vi "SimpleVoltageCurrentCapture.vi"() -> ()   [LabVIEW 2014]
uses:
  <vilib>/Utility/error.llb/DialogType.ctl
  <vilib>/DAQmx/write.llb/DAQmx Write (Analog Wfm 1Chan NSamp).vi
  <vilib>/DAQmx/read.llb/DAQmx Read (Analog 1D Wfm NChan NSamp).vi
  <vilib>/DAQmx/create/channels.llb/DAQmx Create Channel (AI-Voltage-Basic).vi
  <vilib>/DAQmx/configure/timing.llb/DAQmx Timing (Sample Clock).vi
  <vilib>/DAQmx/create/channels.llb/DAQmx Create Channel (AO-Voltage-Basic).vi
  <vilib>/DAQmx/miscellaneous.llb/DAQmx Fill In Error Info.vi
  <vilib>/measure/matone.llb/Extract Single Tone Information 1 Chan.vi
  <vilib>/measure/madcrms.llb/Basic Averaged DC-RMS for 1 Chan.vi
  <vilib>/addons/Electrical Power/Basic/Measurement/Power (1 Channel).vi
  <vilib>/imath/engines/lvmath2/RunTimeEngine/Managers/WorkSpace/UID Generator.vi
  <vilib>/imath/engines/lvmath2/RunTimeEngine/BuiltInFunctions/abs/NIMS_abs(signed).vi
  <instcachedir>/0/NIMS_abs(signed)_C4FCB8E6058B49B797C7C8D53CA5F6EC.lvgen/NIMS_abs(signed)_C4FCB8E6058B49B797C7C8D53CA5F6EC_000.vi
  <vilib>/imath/engines/lvmath2/RunTimeEngine/RunTimeType/NIMS_RunTimeType_From StrictType (excl LVString).vi
  <instcachedir>/0/NIMS_RunTimeType_From StrictType (excl LVString)_15A5391EEA9C4AACB9955AC755B83D29.lvgen/NIMS_RunTimeType_From StrictType (excl LVString)_15A5391EEA9C4AACB9955AC755B83D29_000.vi
  <vilib>/imath/engines/lvmath2/RunTimeEngine/LocalVariableDefStatement/MC_LocalVariableDefStatement_Display.vi
  <vilib>/imath/engines/lvmath2/RunTimeEngine/Managers/SymbolTable/Clear UID.vi
  <vilib>/imath/engines/lvmath2/RunTimeEngine/NodeEndStatement/NIMS_NodeEndStatement_Output.vi
  <instcachedir>/0/NIMS_NodeEndStatement_Output_53EC0D466D134D7ABD903AC30B43404B.lvgen/NIMS_NodeEndStatement_Output_53EC0D466D134D7ABD903AC30B43404B_001.vi
  <vilib>/imath/engines/lvmath2/RunTimeEngine/ErrorHandling/NIMS_Finalize Error.vi
  <vilib>/measure/NI_MAPro.lvlib
  <resource>/objmgr/daqmx.rc
  <vilib>/imath/engines/lvmath2/RunTimeEngine/Managers/SymbolTable/NIMS_WorkSpace.lvlib
  <vilib>/Analysis/NI_AALPro.lvlib
  <vilib>/addons/Electrical Power/Basic/NI_EP_Basic.lvlib
panel:
  out "Numeric":i32
  out "output":waveform(dbl)(graph)={"t0"=timestamp(329.7 s since 1904-01-01), "dt"=0.0001, "Y"=array[998 elements]}
  in  "Triger Pulse":bool
  out "real pulse duration":dbl=0.0005
  in  "Pulse Amplitude":dbl=5.0
  in  "Pulse Duration (s)":dbl=0.0005
  out "Pulse":bool
  out "External Command":string="{ \"command\" : \"ac_v\", \"value\" : 0.0 }\n"
  out "TCP Control":bool
  in  "TCP command in port":u16=37086
  out "IV read duration actual (ms)":dbl=96.66666666666667
  out "IV read duration (ms)":dbl=100.0
  in  "Electrode mode":bool
  out "TCP ADC":bool
  out "Last Transmited Loop Id":i32=-1
  out "Read Loop Id":i32=3296
  out "AC Voltage":dbl=0.015165725599678053 format="%0.2p"
  out "AC Current":dbl=0.0011066504587498834 format="%0.2p"
  in  "TCP data out port":u16=37085
  out "AC I_in amplitude chart":dbl(graph)=0.0011066504587498834
  out "I_in RMS":dbl(graph)=19.597394261114836
  out "Power plot":dbl(graph)=-1.7020442408267042
  out "Phase difference plot":dbl(graph)=291.4389580733613
  out "I _in Power Spectrum":T1(graph)={0.0, "df"=10.000000000000007, "Power Spectrum (V^2 rms)"=[384.05781864212213, 1.2812941664551393e-08, 1.2802014188361118e-07, 4.812511296015439e-09, 3.4604865493181385e-09, 8.59844797514965e-08, 1.540100486406839e-08, 2.7635332673585536e-08, 2.0089632622951103e-07, 2.5397753546698656e-08, 3.0209073625980115e-08, 5.243292855206259e-08, 2.7564168394443787e-08, 1.3099304476836114e-08, 1.0159404130224844e-07, 8.76543417641275e-09, 2.276381425075035e-08, 4.6904899271181916e-09, 9.941137463137335e-09, 1.2446977421983896e-08, 8.579209932008616e-08, 2.0104817814097586e-10, 1.8991275344229937e-08, 9.837888338792514e-08, 6.481034062706947e-08, 7.925498497472071e-08, 7.731911747461447e-08, 1.5782095489234225e-09, 3.279570790933137e-08, 1.349939768318964e-07, 9.63615092297605e-09, 2.9275372363938947e-08, 1.3176389712752455e-07, 4.018791844757954e-08, 3.8489049210479654e-08, 3.209664549280304e-08, 6.31520653319137e-08, 1.062910830558792e-07, 9.767664666009403e-08, 3.7143944529906357e-09, 8.1056328458131e-09, 5.178062053483344e-08, 5.679670399970084e-08, 1.907727598794696e-08, 9.69946931205068e-09, 3.5621842812701156e-08, 3.555275859885974e-08, 1.99230098156712e-07, 5.369362919485012e-08, 4.1863615058039905e-08, 1.2338652677581583e-08, 4.697281997314641e-08, 3.993580605238427e-08, 1.70035079391051e-08, 1.6594795089805326e-08, 1.516958186684704e-07, 7.575946548396981e-08, 2.5612321514999438e-08, 5.2738297712080446e-08, 1.1590760683173937e-07, 2.0944189064547272e-08, 1.0264229746821111e-07, 6.978167227192961e-08, 1.1508175740867062e-07, 8.093287052603338e-08, 3.1301731540051725e-08, 1.454693917268169e-08, 2.9108329285014653e-08, 2.409433105650876e-07, 3.459793455758188e-08, 7.532687221251975e-09, 1.2005768049469254e-08, 4.634528439936204e-08, 1.6745745681336807e-08, 6.172958760008946e-08, 9.655445431991258e-08, 2.4918781782308413e-08, 1.3380696016198607e-08, 9.273295644922437e-09, 9.384676050914868e-09, 5.045622969104436e-08, 1.328983752516565e-07, 1.1221780541437274e-07, 4.141449358779783e-08, 2.903977936074104e-08, 3.8537967200709724e-09, 4.708037887736474e-08, 8.291494602872388e-08, 7.70570911232849e-08, 1.966098960787566e-07, 4.534805900984656e-09, 1.726199435323091e-08, 3.3680113687564556e-08, 1.3805146619739584e-08, 3.472836601578071e-08, 2.630915209312157e-08, 8.168496626292698e-08, 5.0623868146713205e-09, 1.115875074934071e-07, 1.7741127446006096e-07, 4.368995406929392e-08, 3.2021447596937008e-09, 3.48779398152876e-08, 3.081985764940028e-08, 1.1096457286070956e-07, 4.60849417995993e-08, 3.779434226378727e-08, 4.347888166225807e-08, 1.6373452915251257e-09, 1.8808612179755276e-08, 7.988124958811374e-08, 4.376230558771452e-09, 3.339685828609752e-08, 1.0891895570542552e-07, 4.1536321590750644e-08, 4.8098653195030446e-08, 4.6601247081840685e-08, 8.391058107643042e-08, 1.0431839897374635e-08, 1.5214232021995607e-08, 1.8688923087010836e-07, 8.659765798597669e-08, 1.4491551422316902e-07, 2.141816801173361e-08, 1.2072901470805195e-09, 6.3913451504969056e-09, 2.2794143843174313e-08, 8.064368559082834e-08, 1.915399388627138e-07, 1.206705846213626e-08, 4.033054884196688e-09, 2.1342371658332653e-09, 6.075018915623819e-08, 1.4852245888680382e-07, 4.88419660733143e-09, 4.088409395652448e-08, 1.4026863668695995e-07, 2.2252630941062042e-07, 3.5832058304485996e-08, 2.3936499810289502e-08, 2.9039314574844087e-09, 2.3973293286931087e-08, 1.5836479233915926e-07, 2.23325561613219e-08, 1.696949460470778e-08, 8.26262872042607e-09, 6.50783217445291e-08, 1.0775111733297002e-08, 1.0390218139538638e-08, 1.3560599946394992e-08, 5.206753303012184e-08, 4.773172547667066e-09, 1.4873562740571618e-08, 1.9868712281171172e-08, 2.0981036336581242e-09, 8.945525119636087e-09, 4.0189259502991666e-08, 3.952424418931359e-08, 2.894034445292779e-08, 4.6490878327638985e-08, 4.524556389012339e-08, 1.2629162546160513e-09, 2.708985273619554e-08, 1.0223761490440988e-07, 3.594586961713648e-08, 3.5426269882768174e-08, 4.137147998757457e-08, 2.9552957073705045e-08, 2.3365565701057763e-08, 9.26388932893052e-08, 1.1109103449455194e-07, 3.409307933526586e-09, 1.2146773701920775e-07, 4.584882861390524e-08, 9.354375969972158e-08, 1.4321296597243922e-08, 5.977699519636451e-08, 5.9461219291895514e-08, 4.215040396774052e-08, 1.728463184328385e-08, 3.136769765310978e-08, 3.4377428728288975e-08, 4.8818253276382846e-08, 1.7013235743670174e-09, 9.447022422313127e-08, 5.75966470002399e-08, 1.127651177182249e-08, 7.27729417865729e-08, 1.856704451103715e-08, 4.948908503771827e-08, 1.983889196727655e-08, 5.10381999791832e-09, 1.5679008689252454e-08, 2.1741073758842818e-08, 3.7297112056119515e-08, 7.661161766255485e-08, 6.433430558102816e-08, 1.2813926302545611e-08, 3.600763990317574e-07, 1.4561070888716884e-08, 4.949647036914003e-08, 8.129625906523154e-08, 2.9420403092238935e-09, 5.554047301193506e-09, 1.7827901643730115e-08, 1.504997723559743e-08, 1.5023578029496108e-07, 1.4670282386484361e-08, 2.28388341349861e-07, 2.5117787388135496e-08, 2.740953183198227e-08, 5.497198046704744e-08, 4.362641518031774e-08, 4.237109609144519e-08, 3.2688284362417267e-08, 2.5498427822612962e-08, 1.2520509050448536e-07, 2.233767041481571e-08, 3.2941470086808166e-08, 7.455358270842485e-09, 6.632980299635733e-08, 5.90896912581073e-08, 1.5304394394886514e-08, 5.3934963622971515e-08, 3.2767245686984146e-08, 9.612385712461888e-08, 4.8826354287495546e-08, 1.240211384939601e-07, 1.1460957546451582e-07, 2.4898905168286042e-09, 1.772980921047333e-08, 1.2385457753213336e-08, 4.9078691491580206e-08, 3.278255307059739e-08, 3.750081644919358e-09, 1.3931200494654658e-08, 5.444352857635511e-08, 6.546747175751133e-08, 1.711208662881434e-08, 1.929493601896497e-08, 3.6398341900996806e-08, 4.2966173465561364e-08, 3.6755869616760876e-08, 3.0176788219327757e-09, 3.011950207355472e-08, 3.512689585829536e-08, 2.8423326392118875e-08, 1.0022518357393645e-07, 1.4680561564719452e-08, 3.649625294637584e-08, 4.031497162692909e-08, 3.212272725614469e-08, 1.2139641391960006e-09, 7.021303894753625e-08, 3.3063149986789023e-09, 1.2393920457988236e-08, 1.0791191385073534e-08, 9.053090999153262e-08, 1.319342590437711e-07, 1.4614565189317268e-07, 1.5278657963461335e-10, 4.5527749043547795e-08, 1.452004595136674e-07, 1.664928120564626e-08, 5.140611957930399e-09, 7.727909612291312e-09, 1.6165225384853362e-08, 6.759152536161556e-08, 1.6398993135795582e-07, 5.630261658395028e-09, 2.5996461043004046e-08, 7.226217514336062e-09, 2.9198395761224226e-08, 4.306174983650763e-08, 7.004299924871136e-08, 3.519309319534001e-09, 2.91242462930489e-08, 7.060805187155125e-08, 8.056344362369779e-08, 6.180589372203309e-08, 6.940038681131413e-08, 1.1166596987411668e-08, 6.924308293151698e-08, 7.001606609260729e-08, 8.224478674786695e-08, 1.3951863080363851e-08, 2.1019018313440102e-08, 6.907251718509267e-08, 5.681299872508286e-09, 1.7677978248220832e-08, 2.6384605682949153e-08, 6.974791105187748e-09, 8.744045551935272e-08, 6.245895633033074e-08, 2.3706613961085087e-08, 5.624962818699386e-08, 2.8832627632170862e-08, 1.042337329119717e-09, 2.5334040670312715e-08, 2.434183685492577e-08, 7.86786715205878e-09, 1.6131885884860795e-08, 9.67930212416229e-08, 8.995733591895769e-08, 3.593948638488143e-08, 1.2541696411160845e-08, 9.554155040825989e-08, 1.7212725928829574e-08, 4.339613421388269e-08, 1.4565190207604182e-08, 7.578403908246223e-08, 3.723807576887632e-08, 2.2365903775075548e-08, 9.856433197334754e-09, 1.2901973481063502e-09, 3.237236539707619e-08, 1.3401762776921863e-08, 4.28802900320129e-08, 1.009290130906903e-07, 1.1396783394352265e-08, 2.531839857522575e-09, 4.3163400538895804e-08, 8.202540043777047e-08, 8.05816149377029e-09, 1.993864670886027e-08, 1.3644193500555042e-08, 1.3710128091232536e-07, 1.2638350417317973e-07, 5.7553454709946467e-08, 2.5779488948016492e-08, 3.547853169452205e-08, 1.927531482405474e-08, 2.1686066535790113e-08, 5.705752181882103e-08, 3.872519367448343e-08, 2.5710443279786668e-08, 2.745824248594476e-08, 1.0053202733111108e-08, 1.420870517456479e-07, 1.3291045114345208e-07, 1.5089874386483102e-08, 1.3383166408501238e-08, 4.7639242285258216e-08, 4.2779638261412625e-08, 3.5198664594141145e-08, 4.70674751344519e-08, 1.5640362866699093e-08, 2.777259741109804e-08, 1.8464546583383468e-07, 3.5526622377151104e-08, 6.992173052859764e-08, 7.04500361147302e-08, 2.317990914179313e-07, 8.160084189023287e-08, 3.800938308072212e-08, 9.045009934960116e-08, 1.2123057541864966e-07, 9.378510145173343e-09, 9.410955336235093e-08, 3.263838524099404e-08, 3.5637629667962905e-09, 4.77995455931702e-08, 5.368568140428507e-08, 1.322668580298105e-07, 1.0525664473288381e-08, 4.2409000894338724e-08, 1.1913821826190874e-07, 3.6223643278452168e-09, 2.9364053248634797e-08, 6.802727007201526e-08, 2.4686475295655384e-08, 1.3865394342703764e-07, 7.448398837323908e-08, 3.088265147226928e-08, 8.276128342601035e-08, 2.8119971146810945e-09, 6.5311068330998e-08, 8.246058705122179e-08, 1.9612968776879275e-07, 8.688316194537927e-08, 1.0572137449711188e-07, 1.4978541326265806e-08, 7.220451672668149e-09, 3.539964837407443e-08, 4.508792174056677e-08, 1.667337014738283e-08, 7.250899914777877e-08, 6.79692735908802e-08, 2.640801847008435e-08, 8.403841705833863e-09, 3.368100306159142e-08, 4.9455949186695094e-09, 9.330160576087414e-08, 9.1280438659868e-09, 6.971658854059668e-08, 1.9278804379235124e-08, 8.85741070762139e-09, 6.550471987073927e-08, 3.820630276229358e-08, 2.687291584215985e-08, 2.3908490507636175e-08, 2.321404069218755e-08, 3.2214778162993593e-08, 4.388028386243561e-08, 1.2882393967833918e-08, 6.7536187752439464e-09, 1.1744915357741611e-07, 7.18914884229133e-08, 1.9895175149726103e-07, 3.2400929572333717e-09, 9.297016272154701e-08, 9.934642824917249e-08, 8.321767937785236e-08, 5.670142195274526e-08, 4.951672860997498e-08, 1.8452713170003762e-08, 5.4116149816271593e-08, 2.0809817958948804e-08, 2.6881821288426383e-08, 2.1190492285073913e-08, 5.47989710922767e-08, 4.578562112689227e-08, 5.334322628142155e-08, 2.48547407773874e-08, 6.866572229520074e-09, 7.3369066098468025e-09, 1.1056786439640651e-08, 3.2700412463793237e-09, 2.0075139460641065e-08, 2.3881469546759143e-08, 8.966300203801532e-09, 1.2809432909660115e-07, 3.331679010715642e-08, 4.306759826704191e-08, 1.2583136041369329e-08, 7.012631803409424e-09, 4.3090819051484345e-09, 4.1692195154994595e-08, 2.6816404245670878e-08, 2.055791968326877e-09, 1.3672465345410637e-08, 2.1322010842748506e-08, 1.7596748428903714e-07, 4.4949830972338244e-08, 1.0341561615247105e-09, 2.9084161413310027e-08, 5.374387988786714e-08, 5.3349698825652904e-08, 1.4128611673613282e-09, 3.8801402600612375e-08, 3.109126241976239e-08, 3.1098370373565677e-10, 2.926361272648796e-08, 1.0898175300612959e-07, 4.075335025512814e-08, 1.335596727884363e-08, 1.062338525009548e-07, 3.232462556489928e-08, 8.387463408086883e-08, 1.2095210893322399e-08, 5.45334503104955e-08, 6.993509675464793e-08, 1.5871236299946294e-08, 2.706339141278551e-08, 3.0075189364169905e-09, 1.0028254063447421e-07, 3.277337661996945e-08, 5.1868628358504955e-08, 9.293476084725768e-08, 9.769168343283154e-09, 2.706819927179853e-08, 2.4966227555830077e-08, 8.834113407472588e-08, 6.397827295092539e-08, 8.372402954614174e-08, 8.712366376138589e-08, 7.078032696757265e-08, 2.7721920832500157e-08, 2.0649870212633134e-08, 2.5616407575308477e-08, 3.630868795735885e-08, 5.3707571062058424e-08, 8.275253292117417e-08, 1.2025549414428655e-08, 2.816125366723839e-08, 1.9186971038008822e-08, 3.6065289353871736e-11, 3.077636615403747e-09, 1.2370255816695734e-08, 1.0754168043709105e-07, 1.2675781071772376e-08, 2.898987401047185e-08, 4.473663379246382e-09, 3.3432293379785746e-08, 4.291579540032761e-08, 2.4535696702101412e-08, 1.7904473506491875e-08, 1.2969337345251354e-08, 3.579713233883194e-08, 8.306977329479662e-09, 1.1878600002587436e-08, 4.559792218223604e-11, 8.669398160192331e-08, 1.5443681894492246e-08, 5.7040102798961895e-08, 1.5455294911454466e-07, 2.2609903226912203e-08, 3.433387559706304e-08, 3.5888217413332686e-08, 1.941087982577279e-09, 2.7888395771837493e-08, 1.3803208628908935e-08, 4.9739989771947375e-08, 6.56012888081166e-09, 2.6591919552228713e-09, 6.630477591387785e-08, 1.3514257595649928e-07, 8.873512189501864e-09, 5.383031118323386e-09, 4.5274595599770835e-08, 1.2447679041540927e-07, 4.0434634444370015e-08, 6.3588242155244805e-09, 4.11760048095076e-09, 4.268369816964896e-09, 3.3258099950921486e-08, 2.6777423955798133e-08, 1.4054579830603142e-08, 1.156496532066109e-07, 3.395223102219717e-08, 6.230963112132895e-09, 1.3417625574245126e-08, 2.393050690932955e-07, 9.312228370000481e-09, 1.522541587312519e-08, 1.699491322214352e-08, 1.458984318693044e-07, 1.4460492208640573e-08, 1.835723265304928e-08, 2.3116603349858304e-08, 2.289455799857778e-08, 5.494128163325584e-09, 1.2559273977983916e-09, 8.723516991111303e-09, 9.56016883450206e-10, 1.5131137297979946e-08, 3.522116163379456e-08, 1.2780902906619467e-08, 2.0521225464484514e-08, 4.9710476866549016e-08, 2.6723133698770964e-09, 6.611761157113771e-08, 2.17822791711475e-07, 3.529362622749032e-08, 3.559740380027698e-08, 3.0236899652022443e-08, 9.880896042276115e-09, 1.653928219393416e-08, 2.2042260585923302e-08, 1.2119349725733237e-09, 4.263896438113567e-08, 5.9149398327904576e-08, 1.8856320402723333e-09, 2.281966109681429e-08, 5.754600253341904e-08, 5.0430552608468136e-08, 7.281465448753168e-09, 1.0395847299244066e-07, 1.924722587487483e-09, 1.695799004691539e-08, 2.6679578279876708e-08, 8.867086963010186e-09, 3.9524439443566215e-08, 1.1091448657235346e-07, 4.190708095098228e-09, 9.657150920733476e-08, 5.668301325774216e-09, 6.786300981728324e-08, 1.3223520082514987e-08, 3.404814354670106e-08, 4.223834658514782e-08, 3.8092545585383834e-08, 2.9289426487155407e-08, 1.0530287208659933e-09, 1.131762267293828e-09, 4.114102244117353e-08, 7.427298812970256e-09, 7.994081603306406e-08, 2.307637249031202e-07, 8.47724353652218e-09, 6.847887534885516e-08, 3.770997494988641e-08, 6.376403576558253e-08, 7.673744978583936e-09, 3.0838536546473044e-09, 4.700581307275506e-08, 1.3697280597830137e-07, 1.1261535051452766e-08, 5.3237899849287214e-08, 1.3605562050271097e-08, 2.2632883810616355e-08, 3.467444062765444e-08, 9.684926131445288e-08, 1.0635383763208542e-08, 4.356006403351025e-08, 2.2292295215612967e-07, 2.9470228128304294e-08, 2.875211386257933e-08, 2.041494292362725e-07, 6.39615845040027e-08, 5.977660555367681e-09, 6.26720749668346e-09, 5.984571161881243e-08, 1.2241633622245034e-07, 4.039287306691826e-08, 5.467584915815582e-09, 4.927474715376204e-08, 9.735781985113371e-08, 1.3217509024118545e-08, 3.3687734175546405e-08, 1.0542365775903405e-07, 4.517158944115068e-09, 9.726950682807576e-08, 2.387697232191287e-08, 2.7575186808995993e-08, 4.6071486658325546e-08, 8.41553900421575e-09, 1.6977322771610884e-08, 1.097823680664256e-07, 6.098758529615711e-09, 6.257708163733645e-08, 3.3555986343451286e-09, 8.692060193608496e-08, 4.468331572970971e-08, 6.390357629481517e-09, 2.6259264712257616e-08, 6.6745767634947644e-09, 3.587115148670567e-08, 3.523706140447217e-08, 4.126006093083413e-08, 2.4398341308567406e-08, 2.840067155681719e-09, 6.614688931874879e-09, 6.978648377097303e-08, 1.1478053355986801e-07, 4.073691886026624e-08, 6.4493241299896534e-09, 3.7683440704147226e-08, 3.0846089194508202e-09, 1.8048287772729807e-08, 3.337806676761065e-08, 2.977472660181094e-09, 1.0719164896676073e-07, 3.2536992415786914e-08, 2.2247660177635246e-08, 1.1476736545919476e-07, 2.8933953016947526e-08, 2.064106548584373e-08, 3.7223643656169426e-09, 1.843286134032916e-08, 1.892681922314445e-08, 3.712199947459135e-09, 1.6695753023392334e-08, 3.3218032569735317e-09, 1.6706432251667378e-08, 2.7067232095953743e-08, 3.837805045664525e-08, 1.1619197367608606e-07, 4.9924179949261114e-08, 8.464384625585008e-08, 9.690586418497523e-09, 7.179583796338114e-09, 6.217634841721696e-08, 3.2937274120486434e-08, 6.387779642630158e-08, 1.8470753266750935e-08, 3.5434607470527096e-08, 8.154309779516997e-08, 3.8727475603592855e-08, 1.0199854591655693e-08, 4.2154686318987e-08, 2.3675515842321936e-08, 6.333797743041275e-08, 8.985223681037249e-08, 6.497841644804245e-08, 2.914188943128051e-08, 4.560784310819312e-08, 1.3420003396361156e-08, 2.900222042456837e-08, 5.1518128797144566e-08, 3.0436935461941626e-08, 4.934019455520264e-09, 5.471322364342871e-08, 1.8294146250360306e-08, 1.0414336013540128e-07, 6.09864340420173e-09, 2.92160425235546e-08, 6.33802995592567e-08, 2.3095568168877672e-08, 2.428623669085022e-08, 2.5474306923772344e-08, 1.4080727261370552e-08, 4.5730253266045205e-08, 1.482467936763585e-08, 9.136500270332283e-08, 3.830435326792223e-08, 9.189028310552746e-08, 1.6171056084457597e-08, 2.6566605210262435e-08, 3.561591387341651e-10, 1.1896556157900548e-08, 1.3103660240603911e-08, 9.215464274720214e-08, 5.860820049635159e-09, 1.6596173016718347e-08, 7.999763077500574e-09, 2.754185521944779e-09, 4.64402722896503e-08, 4.2607496442374204e-10, 5.7640684496696686e-09, 2.4692578535470032e-08, 1.0675485918539571e-07, 5.075488929402043e-08, 4.316460162997264e-08, 5.0328599887739335e-09, 1.5668634672419503e-08, 1.0516052118361708e-07, 2.32509591277423e-09, 2.4635165122359574e-09, 1.583375293010504e-08, 6.084983597675616e-08, 2.453644347913616e-08, 4.3701545919628674e-08, 1.9314605782062944e-08, 2.649684168940553e-09, 4.777686684066642e-08, 2.65642672299213e-08, 8.31033371125199e-09, 4.481639519392982e-09, 3.0178667227519526e-08, 2.2981288156274775e-08, 7.140154264778307e-08, 3.4722699769530815e-08, 5.704763715175978e-09, 1.751524211308479e-08, 2.1017087512336967e-08, 1.988870949402694e-09, 4.735352048969542e-08, 1.0184723992817028e-08, 1.0817985812319281e-07, 7.937617084550854e-09, 4.390171603002758e-08, 2.4249724354616005e-08, 6.71845512229682e-09, 2.380422799459253e-08, 3.501038985542707e-09, 8.899732893447905e-09, 7.61403441167404e-09, 1.1723064942209228e-08, 2.2535947445598375e-08, 5.3283341740886406e-08, 9.105882842766771e-08, 3.3729411059946585e-08, 4.3940267301023304e-08, 2.1774650147897275e-08, 1.7759675438106559e-09, 2.3164876314791638e-08, 8.82667737460953e-08, 7.920169590988872e-08, 1.457761286773177e-09, 1.498315248699009e-08, 7.069854837264057e-08, 8.418069222277153e-08, 3.3678870417317805e-08, 3.1637243848242373e-08, 6.397428397409701e-09, 3.460972408839841e-08, 9.55072908342938e-09, 3.855474842185562e-08, 4.822523574453309e-09, 8.576037029797383e-08, 2.216732732464861e-08, 1.0731731417077834e-08, 3.361911636226198e-08, 4.434785797278945e-08, 1.3149154938533514e-07, 7.085277617290867e-08, 1.3224332278328078e-08, 1.9284574364398894e-09, 2.4047033269657476e-08, 1.0768520697283966e-07, 1.7553608393402726e-08, 1.3109152689706874e-07, 2.807246107263378e-08, 1.096355836380659e-07, 3.955468560380751e-09, 3.006742765984348e-08, 4.060701567467407e-08, 2.426992353465244e-08, 4.749588183834099e-08, 3.054592303261189e-08, 5.270269009564928e-08, 1.9402090796816506e-07, 2.5981880696136016e-09, 5.5230500003331466e-08, 4.64428118203972e-08, 2.1409958294161802e-10, 2.288066203188495e-08, 4.9980825755820055e-08, 1.674232052066761e-08, 5.6795402906730866e-08, 4.4322727225029266e-08, 2.0615649731299158e-08, 7.224529568663976e-08, 2.8688147683281023e-08, 3.402929380102517e-08, 3.141634728403987e-08, 1.7358690033472963e-08, 3.133749417697372e-08, 1.0551277143603665e-08, 9.12262312148022e-09, 1.2263549613662365e-07, 7.851780105651865e-09, 3.882878845776116e-08, 1.6315378053715675e-08, 4.51897149442903e-08, 4.781910596707131e-08, 8.756918742205452e-09, 1.1619690170861289e-07, 1.3626447576593534e-08, 1.0466638043043739e-08, 4.481027922250179e-08, 6.619337613530257e-08, 4.891485332269246e-10, 5.021283819602683e-10, 2.8838057047061665e-08, 8.830466536655001e-08, 1.1384736417596889e-08, 7.6499005222322e-08, 2.9832437883927726e-08, 2.417383384128457e-08, 1.0785370136026602e-07, 7.010394634407974e-08, 2.2124162123321894e-09, 5.1773802221779206e-08, 1.3397532270908865e-08, 2.9126431058974736e-08, 4.758678297839971e-09, 1.4859726717958443e-08, 9.579290796896566e-10, 8.382410500470574e-08, 7.080310312553315e-09, 2.7269490700317792e-09, 3.78099506757096e-08, 2.2906553673914697e-08, 4.958157328070189e-08, 1.277758260512456e-07, 1.5496214788254566e-08, 8.399442991850865e-09, 2.0974383688651131e-10, 7.653814131921521e-08, 1.0629574548079339e-07, 2.766875061154353e-07, 4.7209301917957004e-08, 1.1853201114255108e-07, 6.937763799420605e-08, 1.943847211188159e-08, 1.2681629635338865e-08, 7.171993830343981e-08, 7.3958949077661664e-09, 1.580972972534488e-08, 4.987889256805363e-09, 1.5029071415743658e-07, 1.1168613268630692e-07, 4.842068320148151e-08, 2.8670743014069843e-08, 7.552634389872825e-09, 3.55254938629143e-09, 4.690651654555333e-08, 9.617146907054903e-08, 3.94990254100245e-08, 2.7489632549819656e-08, 2.023782404563175e-08, 1.582435662631923e-09, 3.1974873935959875e-08, 7.579308377126686e-08, 2.7394549112873103e-08, 6.670929337086143e-08, 2.2152275059967488e-08, 1.3600706174955887e-08, 8.642822088262854e-09, 1.6107839488244233e-08, 8.781916880881347e-09, 3.097308817856408e-09, 2.4331582751704115e-08, 6.087922156947291e-09, 5.591098530859275e-08, 1.5982979887672207e-08, 9.264901077036059e-09, 2.0318992127978495e-09, 4.7404658141317465e-09, 9.173930614178918e-08, 7.152799793383632e-09, 4.131337501520023e-08, 1.2321417755982251e-08, 7.903663090317008e-09, 7.611818940957837e-09, 7.990165836186578e-09, 8.012796359838227e-08, 2.5157892757339584e-08, 6.415511471668318e-08, 1.243422988770215e-08, 3.49275645642184e-08, 3.863971064859102e-08, 3.1525505084313803e-08, 5.879145668430913e-08, 3.061627893242176e-10, 2.0131851195834646e-08, 1.7290712355540862e-08, 6.655802688588835e-08, 6.867426372189385e-09, 2.175498026467824e-08, 3.005946190978901e-08, 1.0725539817075016e-07, 9.906682015982944e-09, 1.9790589684394564e-08, 8.327225304946475e-10, 4.82468904336366e-08, 7.692639511651834e-09, 3.170008967763013e-08, 3.066931712221607e-08, 3.4791852466532265e-08, 3.10052077096927e-08, 4.901097856833149e-08, 8.408839697239916e-08, 1.418586799530674e-08, 4.7117279291701356e-08, 2.310797157029537e-09, 1.4445746485114266e-08, 6.164582516458707e-08, 2.5586830180460847e-08, 8.43785099374807e-08, 7.356410892271902e-08, 2.1885505924809696e-09, 4.7113911161041374e-08, 4.529500492545696e-08, 7.411155338885586e-08, 1.8176061752414404e-08, 5.47078902877339e-09, 3.892521506606838e-10, 2.374747848250165e-08, 3.062240367602707e-08, 6.296928503327405e-08, 4.056519728153538e-08, 5.6650512775013824e-08, 2.7827017241309587e-09, 4.078240649430459e-08, 3.2910104358428584e-10, 1.0526504712502214e-07, 9.78174397904926e-10, 1.8058767377346493e-08, 1.997747703478305e-09, 4.490674360637365e-08, 1.378005989277269e-08, 1.624907623861366e-07, 3.4692154033791618e-09, 5.161169405968163e-08, 2.285652862117089e-08, 8.639929263472041e-08, 7.931550118063889e-09, 1.4958674207442694e-08, 1.7480323340141855e-08, 7.60715363663814e-09, 2.6841314471108995e-08, 6.105837010272096e-08, 8.853220821608051e-09, 6.405650907048701e-11, 5.1875936854683124e-08, 5.3487242573330204e-08, 3.0559786850250324e-08, 3.981132646282874e-08, 1.8316925521886576e-08, 9.894007164716781e-09, 5.745944411915238e-09, 1.1143621083510306e-07, 6.238823250824436e-08, 5.541522312654942e-08, 4.3326359896416684e-09, 5.566996620276415e-08, 7.342344959134149e-09, 4.6455232860503546e-08, 4.237100632416493e-08, 1.1083885687882875e-08, 3.466333511838009e-08, 1.2120668315412319e-08, 4.6398686364235566e-08, 1.0906465242535382e-07, 1.1452052680285153e-09, 2.2273214276086914e-08, 1.753520472587311e-08]}
  out "phase difference":dbl=291.4389580733613
  out "detected frequency U":dbl=3135.969897018442 format="%.2p"
  out "detected frequency I":dbl=3776.0681138056098 format="%.2p"
  out "Cuurent and Voltage":waveform(dbl)[](graph)=[{"t0"=timestamp(3525370740.881266 s since 1904-01-01), "dt"=4.999999999999997e-05, "Y"=array[2000 elements], "attributes"=variant("NI_ChannelName"=variant(string "DAC/ai0"), "NI_UnitDescription"=variant(string "Volts"))}, {"t0"=timestamp(3525370740.881277 s since 1904-01-01), "dt"=4.999999999999997e-05, "Y"=array[2000 elements], "attributes"=variant("NI_ChannelName"=variant(string "DAC/ai1"), "NI_UnitDescription"=variant(string "Volts"))}]
  in  "Wave On/Off":bool
  in  "V_out":dbl
  out "Pulse generator":waveform(dbl)(graph)={"t0"=timestamp(329.7 s since 1904-01-01), "dt"=0.0001, "Y"=array[998 elements]}
  in  "V_out Units":dbl=0.01
  out "Mode Changed":bool
  out "V_out sampling rate":dbl=10000.0
  in  "Number of Samples":i32=1000
  out "Wave generator":waveform(dbl)(graph)={"t0"=timestamp(329.7 s since 1904-01-01), "dt"=0.0001, "Y"=array[1000 elements]}
  in  "Oscilator\nSettings":T2={"Waveform Type"=0, "Amplitude"=0.0, "Frequency"=50.0} {"Frequency" format="%0.2p"; "Amplitude" format="%0.2p"; "Waveform Type" items=["Sine Wave", "Triangle Wave", "Square Wave", "Sawtooth Wave"]}
  in  "V_out offset auto-calibrate":bool
  in  "V_out scaling auto-calibrate":bool
  in  "V_in scaling":dbl=1.0
  in  "I_in scaling":dbl=1.0
  in  "V_out offset":dbl
  in  "V_out scaling":dbl=1.0
  out "DC I_in Chart":dbl(graph)=19.59739315934959
  out "Closing Program":bool=TRUE
  in  "IV min V":dbl=-50.0
  in  "IV max V":dbl=50.0
  out "IV progress":dbl(slide)=1.0 scale=0.0..1.0
  in  "IV Relaxation Time (ms)":i32=1000 min=2 step=1
  in  "IV Number of Steps":i32=11 min=2 step=1
  in  "Take IV":bool
  out "Gain (alpha*beta)":dbl=0.1
  out "DC Voltage":dbl=-0.08685133420839247 format="%0.2p"
  out "DC Current":dbl=19.59739315934959 format="%0.2p"
  in  "Samples to read":i32=2000
  in  "I_in Units":dbl=1.0 caption="I Measured Scaling"
  in  "V_in Units":dbl=100.0
  in  "STOP":bool
  in  "Sampling frequency":dbl=20000.0 format="%#_6p"
  # "Units: \nVoltage [mV]\nCurrent [nA]"
  # "Configuration"
  # "Unit Config (don't change)"
  # "Calibration"
  # "Hz"
  # "delete?"
  # "TCP connection"
  # "Electrode Mode"
  # "Imaging"
  # "Deposition"
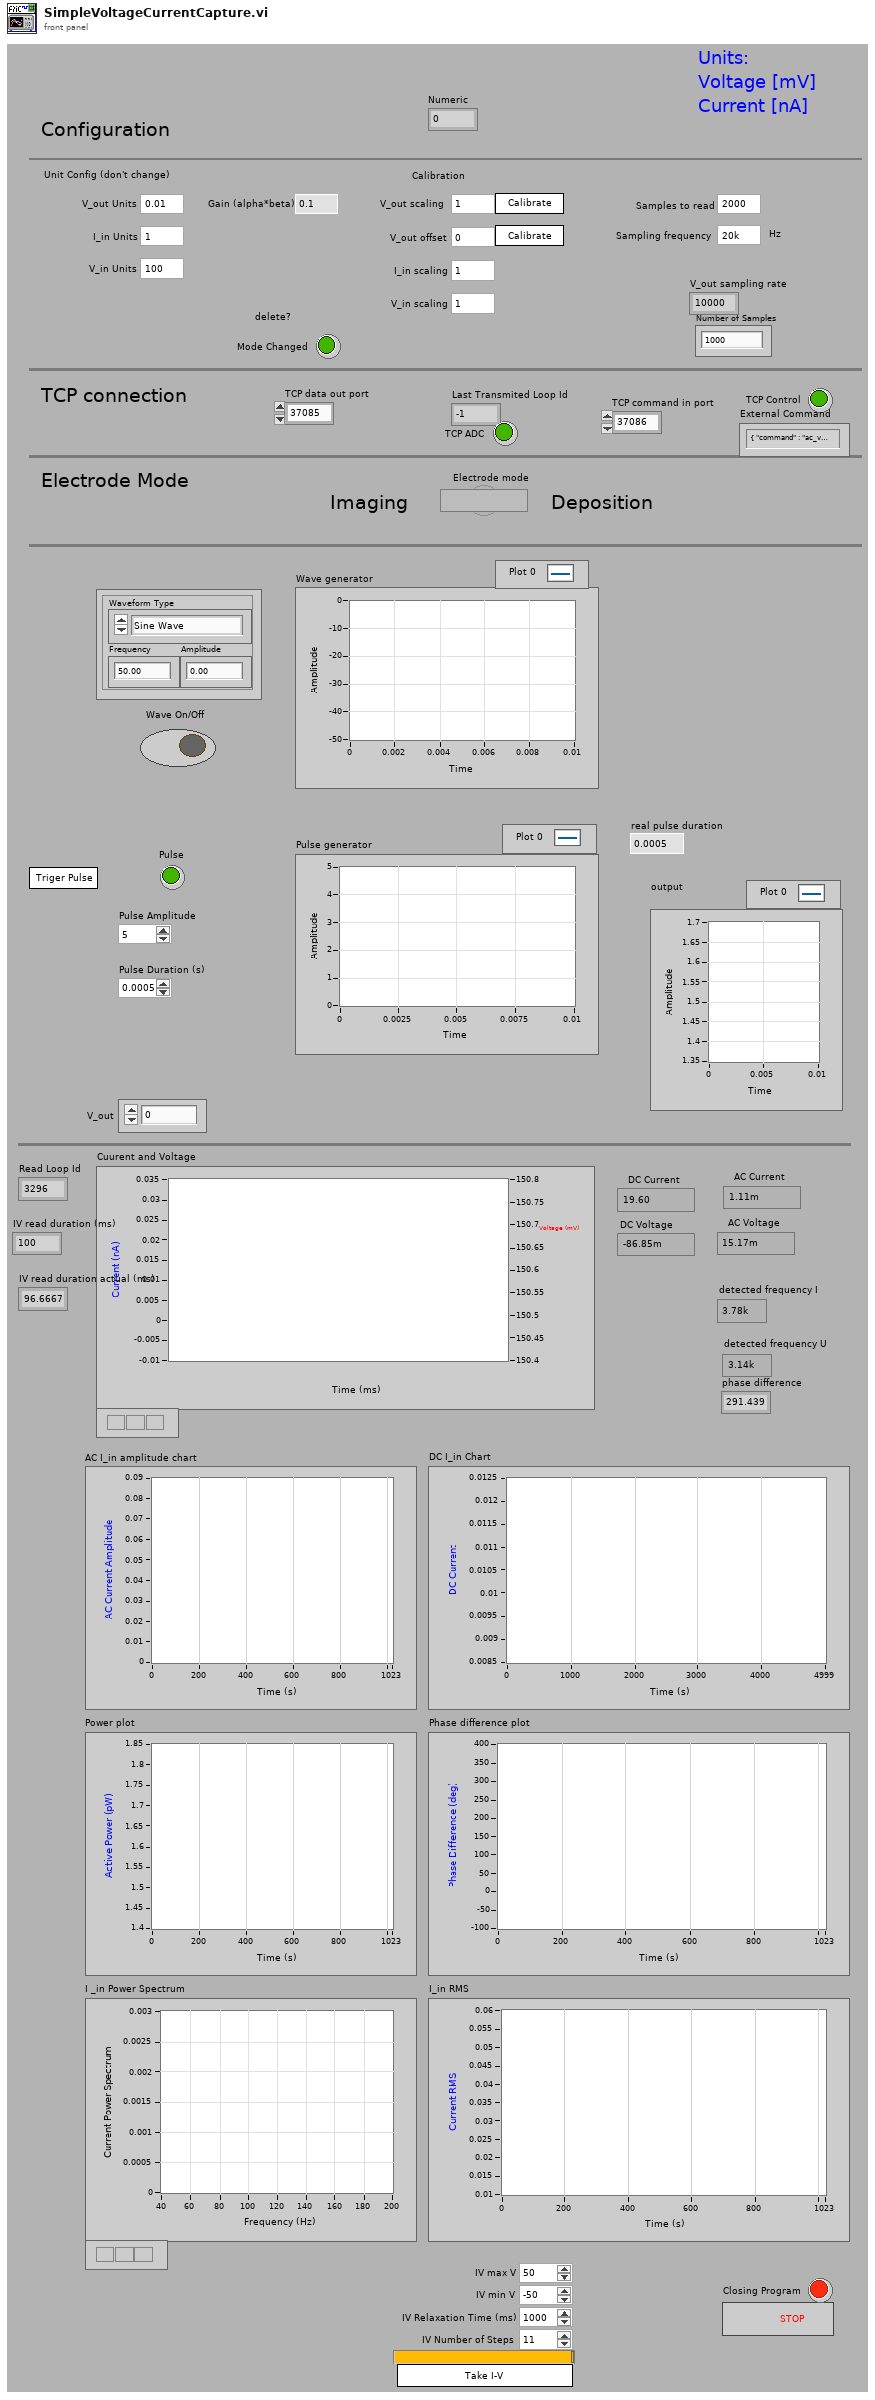
[diagram p1: front panel]
types:
  T1 = cluster{dbl, "df":dbl, "Power Spectrum (V^2 rms)":dbl[]}
  T2 = cluster{"Waveform Type":u16, "Amplitude":dbl, "Frequency":dbl}
  T3 = typedef "DialogType.ctl" = u16
  T4 = typedef "NI_EP_Basic.lvlib/basic_Power Value.ctl" = cluster{"active power [W]":dbl, "apparent power [VA]":dbl, "reactive power [VAR]":dbl, "power factor":dbl}
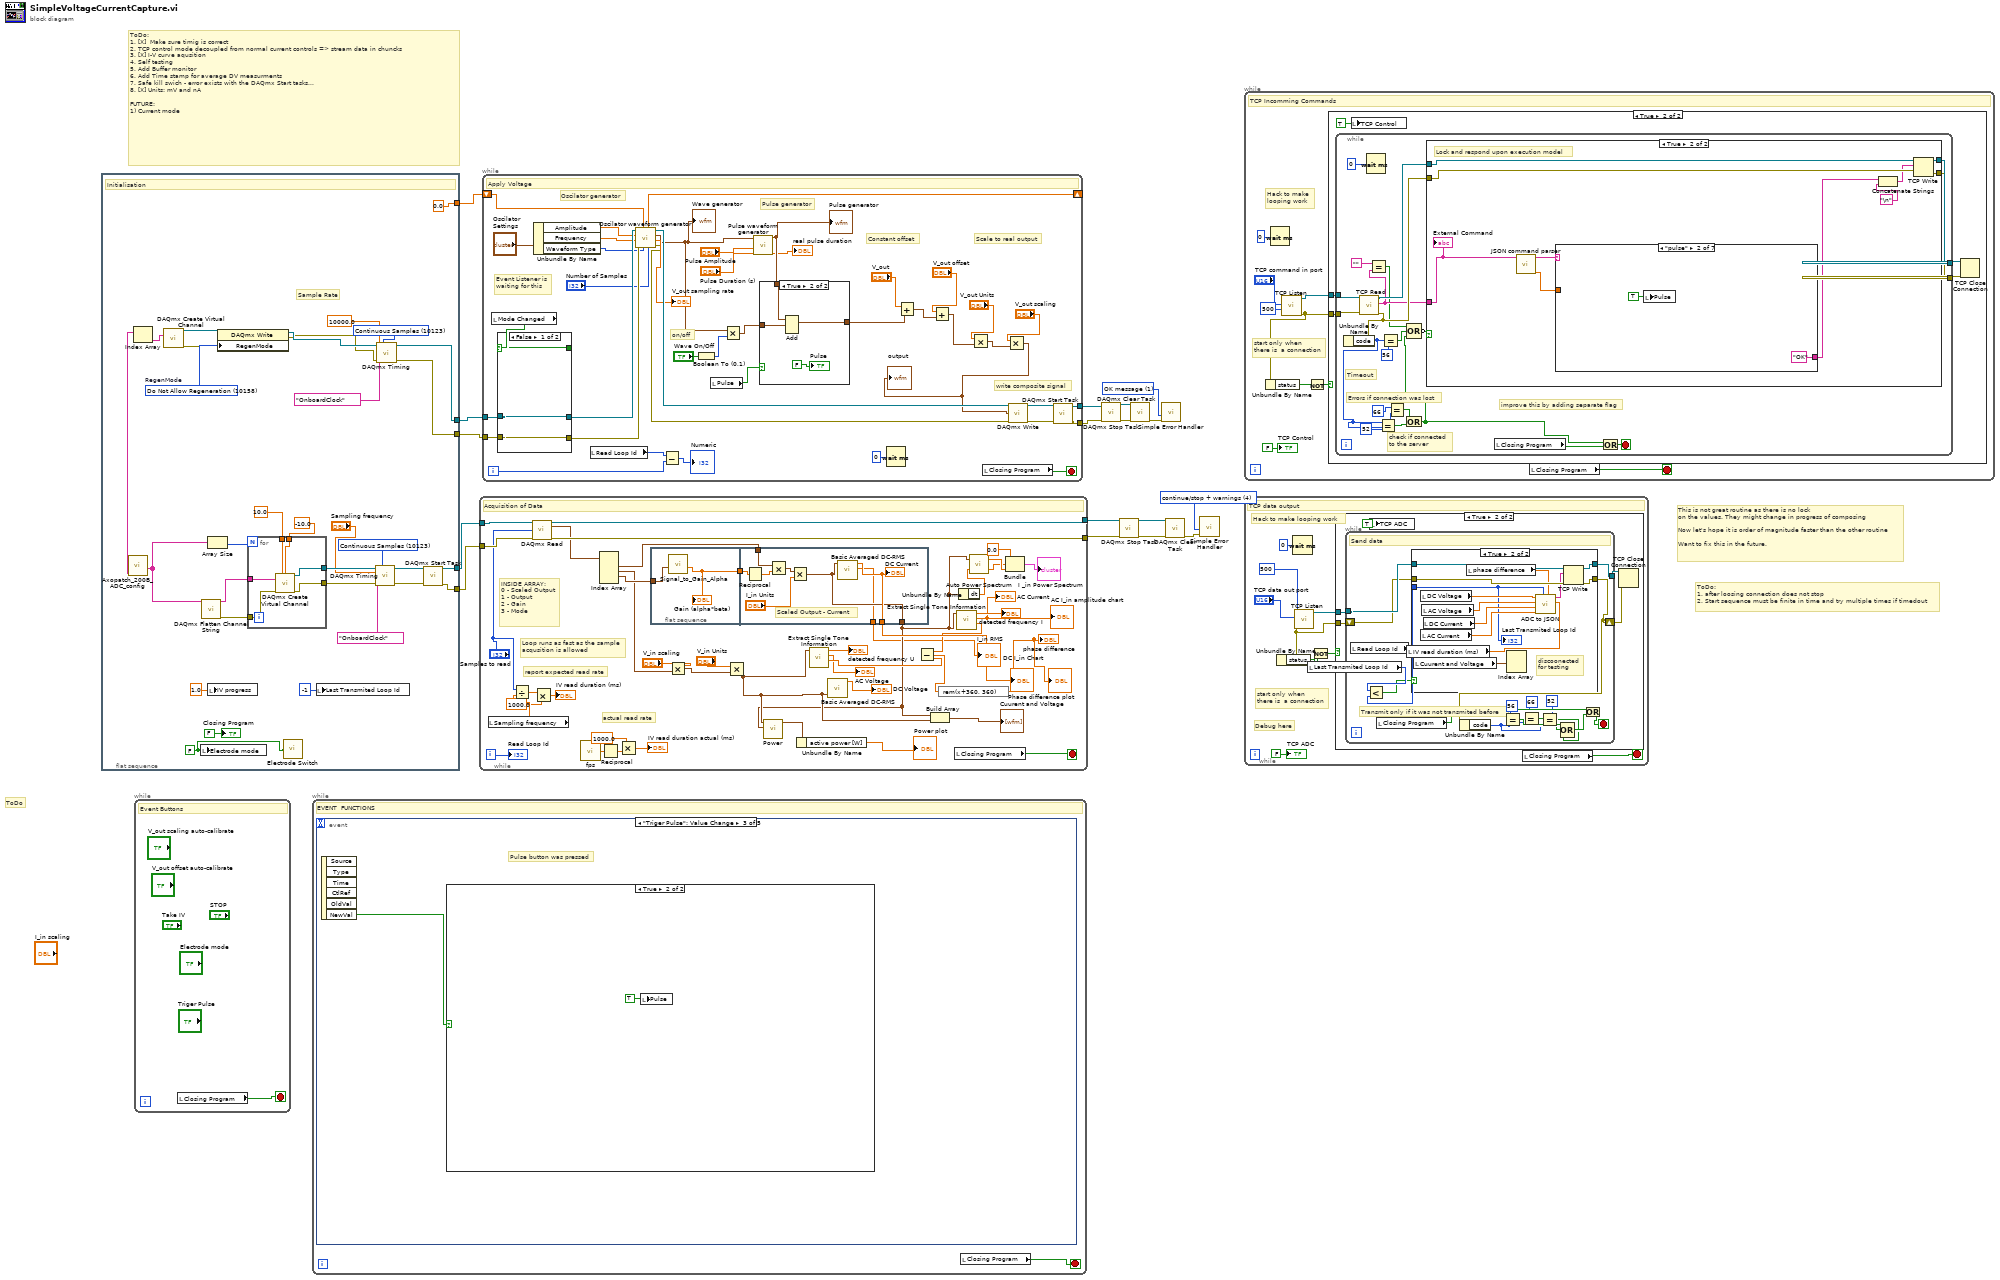
[diagram p0: block diagram]
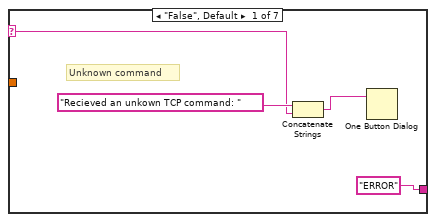
[diagram p4: hidden frame]
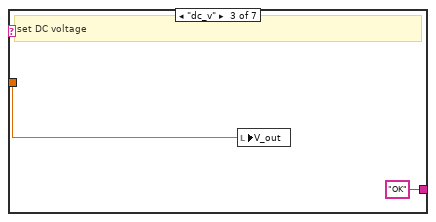
[diagram p5: hidden frame]
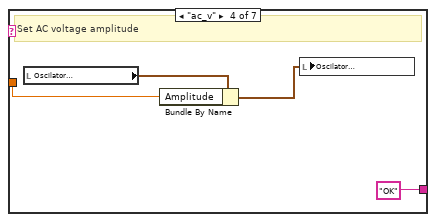
[diagram p6: hidden frame]
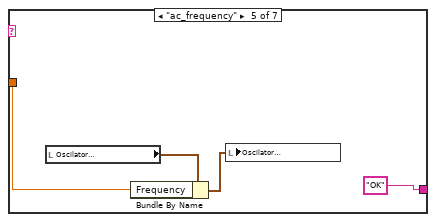
[diagram p7: hidden frame]
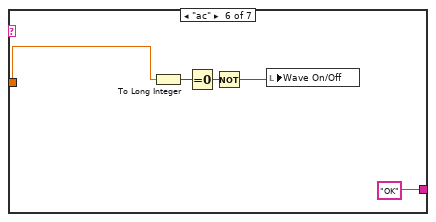
[diagram p8: hidden frame]
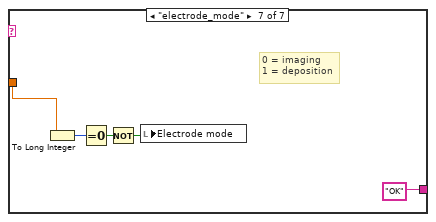
[diagram p9: hidden frame]
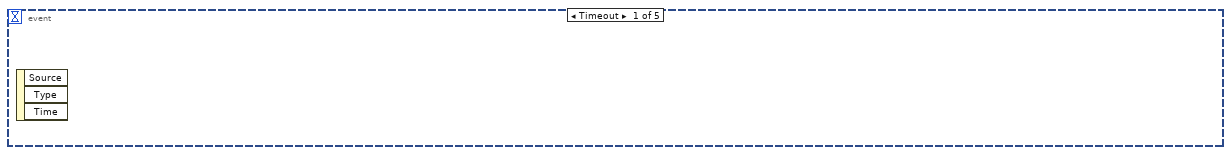
[diagram p12: hidden frame]
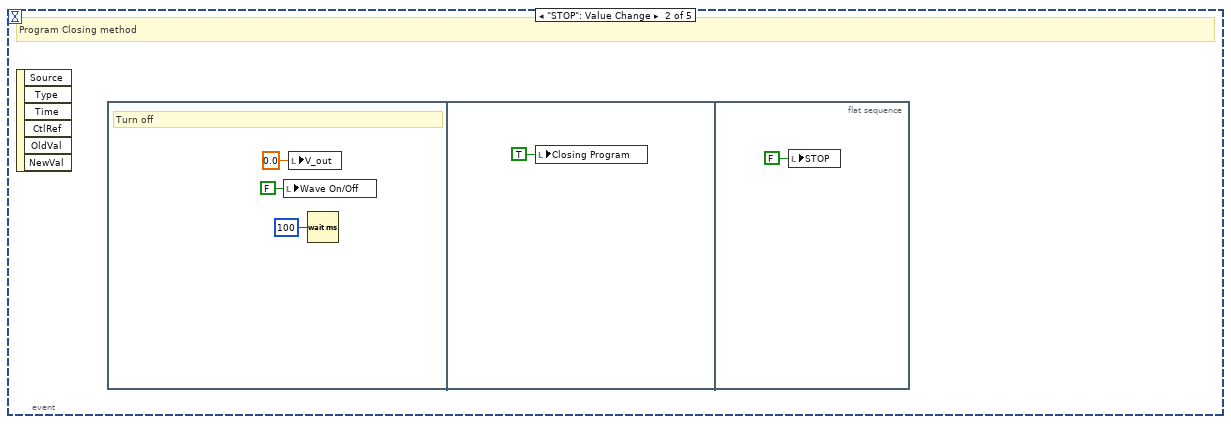
[diagram p13: hidden frame]
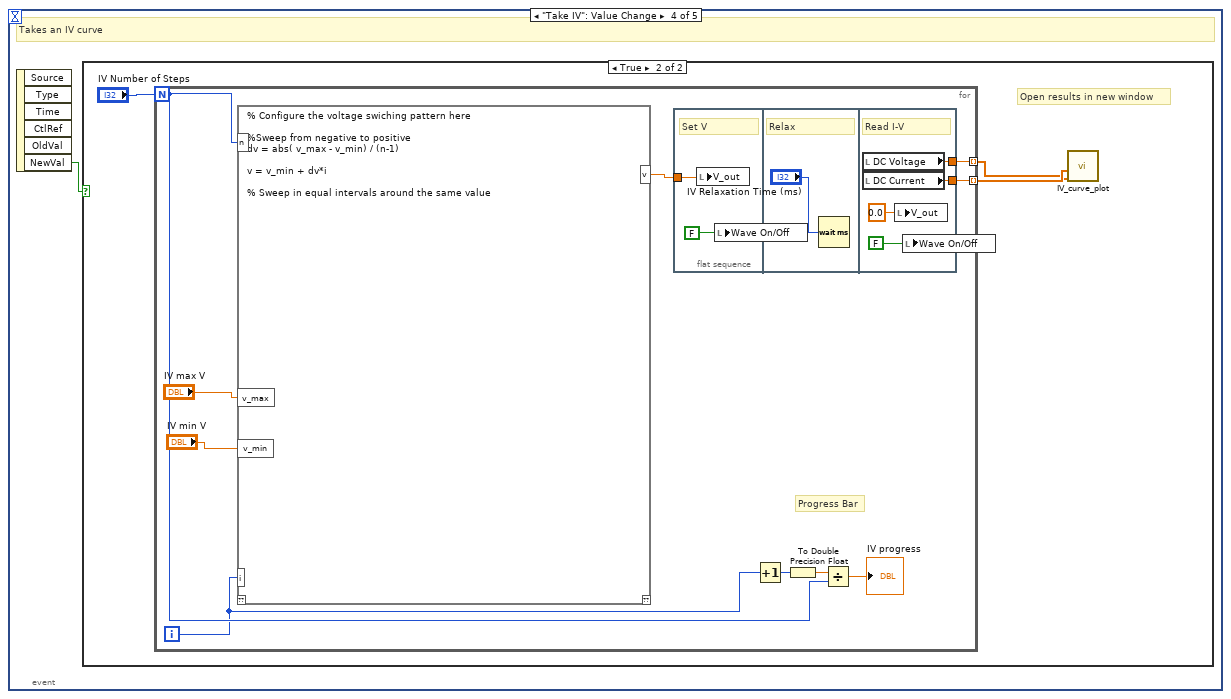
[diagram p15: hidden frame]
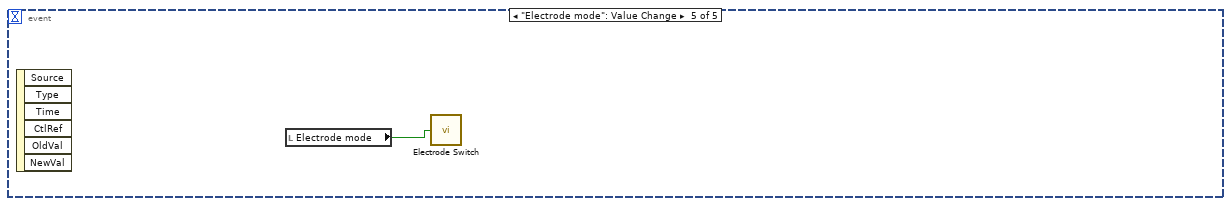
[diagram p17: hidden frame]
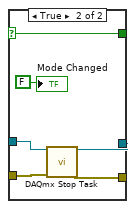
[diagram p19: hidden frame]
diagram:
  w14 = T3 4 items=["no dialog", "OK message", "continue or stop message", "OK message + warnings", "continue/stop + warnings"] ("type of dialog (OK msg:1)")
  w15 = T3 1 items=["no dialog", "OK message", "continue or stop message", "OK message + warnings", "continue/stop + warnings"] ("type of dialog (OK msg:1)")
  # "ToDo:\n1. after loosing connection does not stop\n2. Start sequence must be finite in time and try multiple times if timedout"
  # "This is not great routine as there is no lock\non the values. They might change in progress of composing\n\nNow let's hope it is order of magnitude faster than the other routine\n\nWant to fix this in the future."
  # "ToDo"
  # "ToDo:\n1. [X]  Make sure timig is correct\n2. TCP control mode decoupled from normal current controls => stream data in chuncks\n3. [X] I-V curve aqusition\n4. Self testing\n5. Add Buffer monitor\n6. Add Time stamp for average DV measurments\n7. Safe kill swich - error exists with the DAQmx Start tasks...\n8. [X] Units: mV and nA\n\nFUTURE:\n1) Current mode"
  n1 = flat-sequence {
    tunnel: [w40] -> w17
    tunnel: [w39] -> w16
    tunnel: [w22] -> w12
    tunnel: [w21] -> w11
    tunnel: [0.0] -> w1
    frame #0 {
      w19 = FALSE ("Electrode mode")
      w27 = 10123 items=["Finite Samples"=10178, "Continuous Samples"=10123, "Hardware Timed Single Point"=12522] ("Sample Mode")
      w30 = 10158 items=["Allow Regeneration"=10097, "Do Not Allow Regeneration"=10158]  # RegenMode
      w48 = 10123 items=["Finite Samples"=10178, "Continuous Samples"=10123, "Hardware Timed Single Point"=12522] ("sample mode")
      # "Sample Rate"
      # "Initialisation"
      n2 = call "Axopatch_200B_ADC_config.vi"() -> ("DAC Outputs"=w36:tag[], "DAC Inputs"=w37:tag[])  [unwired: 10 in]
      n3 = Index Array(array=w36) -> (element=w35:tag)  [unwired: 1 in]
      n4 = call-poly <vilib>:"DAQmx Create Virtual Channel.vi"("physical channels"=w35) -> ("task out"=w29:refnum<k21>, "error out"=w28:errorcluster)  [unwired: 13 in]
      n5 = local write "Electrode mode"(w19) -> ()
      n6 = call <vilib>:"DAQmx Flatten Channel String.vi"("names in"=w37) -> ("names out"=w38:string, "error out"=w46:errorcluster)  [unwired: 13 in]
      n7 = local write "IV progress"(1.0 ("IV progress")) -> ()
      n8 = Array Size(array=w37) -> (size(s)=w47:i32)
      n9 = property class="DAQmx Write"(reference=w29, error in=w28, "RegenMode"=w30) -> (reference out=w24:refnum<k21>, error out=w23:errorcluster)
      n10 = for {
        N: w47 -> [_]
        tunnel: w46 -> [w55]
        tunnel: [w54] -> w44
        tunnel: [w53] -> w42
        tunnel: 10.0 ("maximum value") -> [w52]
        tunnel: -10.0 ("maximum value") -> [w51]
        tunnel: w38 -> [w50]
        n11 = call-poly <vilib>:"DAQmx Create Virtual Channel.vi"("maximum value"=w52, "minimum value"=w51, "physical channels"=w50, "error in"=w55) -> ("task out"=w54:refnum<k21>, "error out"=w53:errorcluster)  [unwired: 10 in]
      }
      n12 = call "Electrode Switch.vi"("Electrode F-1 or T-2"=w19) -> ()  [unwired: 3 in]
      n13 = local write "Last Transmited Loop Id"(-1 ("Last Transmited Loop Id")) -> ()
      n14 = call-poly <vilib>:"DAQmx Timing.vi"("task/channels in"=w44, "sample mode"=w48, "rate"="Sampling frequency", "source"=tag "OnboardClock", "error in"=w42) -> ("task out"=w43:refnum<k21>, "error out"=w49:errorcluster)  [unwired: 9 in]
      n15 = call-poly <vilib>:"DAQmx Timing.vi"("task/channels in"=w24, "sample mode"=w27, "rate"=10000.0, "source"=tag "OnboardClock", "error in"=w23) -> ("task out"=w22:refnum<k21>, "error out"=w21:errorcluster)  [unwired: 9 in]
      n16 = call <vilib>:"DAQmx Start Task.vi"("task/channels in"=w43, "error in"=w49) -> ("task out"=w39:refnum<k21>, "error out"=w40:errorcluster)  [unwired: 12 in]
      "Closing Program" <- FALSE ("Closing Program")
    }
  }
  n17 = while {
    stop <- w56 stop-if-true
    # "Event Buttons"
    n18 = local read "Closing Program"() -> (w56:bool)
  }
  n19 = while {
    stop <- w57 stop-if-true
    # "EVENT  FUNCTIONS"
    n20 = event shown="[2] \"Triger Pulse\": Value Change" {
      selector: _ -> [_ _ _ _ _]
      dyn-events: _ -> [_ _ _ _ _]
      timeout: _ -> [_ _ _ _ _]
      event Timeout {
        n21 = event-data() -> ()  [unwired: 1 in, 3 out]
      }
      event "STOP": Value Change {
        # "Program Closing method"
        n22 = event-data() -> ()  [unwired: 1 in, 6 out]
        n23 = flat-sequence {
          frame #0 {
            # "Turn off"
            n24 = local write "Wave On/Off"(FALSE) -> ()
            n25 = local write "V_out"(0.0 ("V Out")) -> ()
            n26 = Wait (ms)(milliseconds to wait=u32 100) -> ()  [unwired: 1 out]
          }
          frame #1 {
            n27 = local write "Closing Program"(TRUE ("Closing Program")) -> ()
          }
          frame #2 {
            n28 = local write "STOP"(FALSE ("STOP")) -> ()
          }
        }
      }
      event "Triger Pulse": Value Change {
        # "Pulse button was pressed"
        n29 = event-data() -> ("NewVal"=w63:bool)  [unwired: 1 in, 5 out]
        n30 = case shown="True" w63 {
          frame False {
          }
          frame True {
            n31 = local write "Pulse"(TRUE ("Pulse")) -> ()
          }
        }
      }
      event "Take IV": Value Change {
        # "Takes an IV curve"
        n32 = event-data() -> ("NewVal"=w65:bool)  [unwired: 1 in, 5 out]
        n33 = case shown="True" w65 {
          frame False {
          }
          frame True {
            # "Open results in new window"
            n34 = for {
              N: "IV Number of Steps" -> [w74]
              tunnel: [w77] -> w66 mode=indexing
              tunnel: [w76] -> w67 mode=indexing
              i -> [w70]
              # "Progress Bar"
              n35 = mathscript code="% Configure the voltage swiching pattern here\n\n%Sweep from negative to positive\ndv = abs( v_max - v_min) / (n-1)\n\nv = v_min + dv*i\n\n% Sweep in equal intervals around the same value"("i"=w70, "v_max"="IV max V", "v_min"="IV min V", "n"=w74) -> ("v"=w78:dbl)  [unwired: 1 in, 1 out]
              n36 = flat-sequence {
                tunnel: w78 -> [w80]
                tunnel: [w85] -> w77
                tunnel: [w84] -> w76
                frame #0 {
                  # "Set V"
                  n37 = local write "V_out"(w80) -> ()
                  n38 = local write "Wave On/Off"(FALSE) -> ()
                }
                frame #1 {
                  # "Relax"
                  n39 = Wait (ms)(milliseconds to wait="IV Relaxation Time (ms)") -> ()  [unwired: 1 out]
                }
                frame #2 {
                  # "Read I-V"
                  n40 = local read "DC Voltage"() -> (w85:dbl)
                  n41 = local read "DC Current"() -> (w84:dbl)
                  n42 = local write "V_out"(0.0 ("V Out")) -> ()
                  n43 = local write "Wave On/Off"(FALSE) -> ()
                }
              }
              n44 = Increment(x=w70) -> (x+1=w69:i32)
              n45 = To Double Precision Float(number=w69) -> (double precision float=w73:dbl)
              n46 = Divide(x=w73, y=w74) -> (x/y=→"IV progress":dbl)
            }
            n47 = call "IV_curve_plot.vi"("I"=w67, "V"=w66) -> ()  [unwired: 7 in, 2 out]
          }
        }
      }
      event "Electrode mode": Value Change {
        n48 = event-data() -> ()  [unwired: 1 in, 6 out]
        n49 = local read "Electrode mode"() -> (w150:bool)
        n50 = call "Electrode Switch.vi"("Electrode F-1 or T-2"=w150) -> ()  [unwired: 3 in]
      }
    }
    n51 = local read "Closing Program"() -> (w57:bool)
  }
  n52 = while {
    tunnel: w17 -> [w194]
    tunnel: w16 -> [w191]
    tunnel: [w193] -> w4
    tunnel: [w192] -> w3
    i -> [w160]
    stop <- w186 stop-if-true
    # "actual read rate"
    # "report expected read rate"
    # "Loop runs as fast as the sample\nacqusition is allowed"
    # "INSIDE ARRAY:\n0 - Scaled Output\n1 - Output\n2 - Gain\n3 - Mode"
    # "Acquisition of Data"
    n53 = local read "Sampling frequency"() -> (w158:dbl)
    n54 = Divide(x="Samples to read", y=w158) -> (x/y=w157:dbl)
    n55 = call-poly <vilib>:"DAQmx Read.vi"("task/channels in"=w191, "number of samples per channel"="Samples to read", "error in"=w194) -> ("task out"=w193:refnum<k21>, "data"=w190:waveform(dbl)[], "error out"=w192:errorcluster)  [unwired: 10 in]
    n56 = Multiply(x=w157, y=1000.0) -> (x*y=→"IV read duration (ms)":dbl)
    n57 = call "fps.vi"() -> ("FPS"=w154:dbl)  [unwired: 1 in]
    n58 = Index Array(array=w190) -> (element #1=w188:waveform(dbl), element #2=w183:waveform(dbl), element #3=w189:waveform(dbl))  [unwired: 4 in, 1 out]
    n59 = Reciprocal(x=w154) -> (1/x=w153:dbl)
    n60 = Multiply(x=1000.0, y=w153) -> (x*y=→"IV read duration actual (ms)":dbl)
    n61 = flat-sequence {
      tunnel: w189 -> [w196]
      tunnel: [w195] -> w187
      tunnel: w188 -> [w204]
      tunnel: w187 -> [w201]
      tunnel: [w199] -> w181
      tunnel: [w198] -> w168
      tunnel: [w197] -> w163
      frame #0 {
        n62 = call "Signal_to_Gain_Alpha.vi"("Gain Signal In"=w196) -> ("Gain (alpha)"=w195:dbl)  [unwired: 10 in]
        "Gain (alpha*beta)" <- w195
      }
      frame #1 {
        # "Scaled Output - Current"
        n63 = Reciprocal(x=w201) -> (1/x=w200:dbl)
        n64 = Multiply(x=w204, y=w200) -> (x*y=w203:waveform(dbl))
        n65 = Multiply(x=w203, y="I_in Units") -> (x*y=w198:waveform(dbl))
        n66 = call-poly <vilib>:"Basic Averaged DC-RMS.vi"("signal in"=w198) -> ("RMS value"=w197:dbl, "DC value"=w199:dbl)  [unwired: 4 in, 5 out]
        "DC Current" <- w199
      }
    }
    n67 = Multiply(x="V_in scaling", y=w183) -> (x*y=w184:waveform(dbl))
    n68 = Multiply(x="V_in Units", y=w184) -> (x*y=w169:waveform(dbl))
    n69 = call-poly <vilib>:"Power.vi"("current waveform"=w168, "voltage waveform"=w169) -> ("power value"=w167:T4)  [unwired: 8 in, 1 out]
    n70 = Unbundle By Name(w167) -> ("active power [W]"=→"Power plot":dbl)
    n71 = call-poly <vilib>:"Extract Single Tone Information.vi"("time signal in"=w169) -> ("detected phase (deg)"=w175:dbl, "detected amplitude"=→"AC Voltage":dbl, "detected frequency"=→"detected frequency U":dbl)  [unwired: 5 in, 3 out]
    n72 = call-poly <vilib>:"Basic Averaged DC-RMS.vi"("signal in"=w169) -> ("DC value"=→"DC Voltage":dbl)  [unwired: 4 in, 6 out]
    n73 = Build Array(w168, w169) -> (→"Cuurent and Voltage":waveform(dbl)[])
    n74 = local read "Closing Program"() -> (w186:bool)
    n75 = call-poly <vilib>:"Extract Single Tone Information.vi"("time signal in"=w168) -> ("detected phase (deg)"=w176:dbl, "detected amplitude"=→"AC I_in amplitude chart" →"AC Current":dbl, "detected frequency"=→"detected frequency I":dbl)  [unwired: 5 in, 3 out]
    n76 = Subtract(x=w176, y=w175) -> (x-y=w166:dbl)
    n77 = expression code="rem(x+360, 360)"(w166) -> (→"phase difference" →"Phase difference plot":dbl)
    n78 = Unbundle By Name(w168) -> ("dt"=w171:dbl)
    n79 = call <vilib>:"Auto Power Spectrum.vi"("dt"=w171, "Signal (V)"=w168) -> ("df"=w173:dbl, "Power Spectrum (V^2 rms)"=w174:dbl[])
    n80 = Bundle(0.0, "df"=w173, "Power Spectrum (V^2 rms)"=w174) -> (→"I _in Power Spectrum":T1)  [unwired: 1 in]
    "DC I_in Chart" <- w181
    "I_in RMS" <- w163
    "Read Loop Id" <- w160
  }
  n81 = while {
    tunnel: w12 -> [w243]
    tunnel: w11 -> [w242]
    tunnel: [w245] -> w7
    tunnel: [w244] -> w6
    shift-right: [w229] -> _
    shift-left: w1 -> [w236]
    i -> [w206]
    stop <- w246 stop-if-true
    # "write composite signal"
    # "Scale to real output"
    # "on/off"
    # "Constant offset"
    # "Pulse generator"
    # "Oscilator generator"
    # "Event Listener is \nwaiting for this"
    # "Apply Voltage"
    n82 = local read "Mode Changed"() -> (w241:bool)
    n83 = case shown="False" w241 {
      selector: w241 -> [w252 w257]
      tunnel: w243 -> [w254 w260]
      tunnel: w242 -> [w253 w259]
      tunnel: [w254 w256] -> w235
      tunnel: [w253 w255] -> w232
      tunnel: [w252 w257] -> _
      frame False {
      }
      frame True {
        n84 = call <vilib>:"DAQmx Stop Task.vi"("task/channels in"=w260, "error in"=w259) -> ("task out"=w256:refnum<k21>, "error out"=w255:errorcluster)  [unwired: 12 in]
        "Mode Changed" <- FALSE ("Mode Changed")
      }
    }
    n85 = Unbundle By Name("Oscilator\nSettings") -> ("Amplitude"=w234:dbl, "Frequency"=w233:dbl, "Waveform Type"=w231:u16)
    n86 = local read "Read Loop Id"() -> (w207:i32)
    n87 = call "Oscilator waveform generator.vi"("Number of Samples"="Number of Samples", "signal type"=w231, "phase in"=w236, "error in"=w232, "Frequency"=w233, "Amplitude"=w234, "DAQdx task in"=w235) -> ("error out"=w213:errorcluster, "MAQdx sampling rate"=→"V_out sampling rate":dbl, "Oscilator waveform"=w223:waveform(dbl), "DAQdx task out"=w228:refnum<k21>, "phase out"=w229:dbl)
    "Wave generator" <- w223
    n88 = Subtract(x=w207, y=w206) -> (x-y=→"Numeric":i32)
    n89 = Boolean To (0,1)(Boolean="Wave On/Off") -> (0, 1=w220:i16)
    n90 = local read "Pulse"() -> (w209:bool)
    n91 = Multiply(x=w223, y=w220) -> (x*y=w222:waveform(dbl))
    n92 = call "Pulse waveform generator.vi"("Base waveform"=w223, "Pulse Amplitude"="Pulse Amplitude", "Pulse Duration"="Pulse Duration (s)") -> ("Pulse waveform"=w226:waveform(dbl), "real pulse duration"=→"real pulse duration":dbl)  [unwired: 6 in]
    "Pulse generator" <- w226
    n93 = case shown="True" w209 {
      tunnel: w226 -> [_ w251]
      tunnel: w222 -> [w247 w250]
      tunnel: [w247 w249] -> w225
      frame False {
      }
      frame True {
        n94 = Add(1:w250, 2:w251) -> (0:w249:waveform(dbl))  [unwired: 1 in, 1 out]
        "Pulse" <- FALSE ("Pulse")
      }
    }
    n95 = Wait (ms)(milliseconds to wait=u32 0) -> ()  [unwired: 1 out]
    n96 = Add(x="V_out", y=w225) -> (x+y=w215:waveform(dbl))
    n97 = Add(x="V_out offset", y=w215) -> (x+y=w214:waveform(dbl))
    n98 = Multiply(x="V_out Units", y=w214) -> (x*y=w218:waveform(dbl))
    n99 = local read "Closing Program"() -> (w246:bool)
    n100 = Multiply(x="V_out scaling", y=w218) -> (x*y=w208:waveform(dbl))
    "output" <- w208
    n101 = call-poly <vilib>:"DAQmx Write.vi"("task/channels in"=w228, "data"=w208, "error in"=w213) -> ("task out"=w238:refnum<k21>, "error out"=w237:errorcluster)  [unwired: 10 in, 1 out]
    n102 = call <vilib>:"DAQmx Start Task.vi"("task/channels in"=w238, "error in"=w237) -> ("task out"=w245:refnum<k21>, "error out"=w244:errorcluster)  [unwired: 12 in]
  }
  n103 = call <vilib>:"DAQmx Stop Task.vi"("task/channels in"=w7, "error in"=w6) -> ("task out"=w9:refnum<k21>, "error out"=w8:errorcluster)  [unwired: 12 in]
  n104 = call <vilib>:"DAQmx Stop Task.vi"("task/channels in"=w4, "error in"=w3) -> ("task out"=w5:refnum<k21>, "error out"=w2:errorcluster)  [unwired: 12 in]
  n105 = call <vilib>:"DAQmx Clear Task.vi"("task in"=w9, "error in"=w8) -> ("error out"=w10:errorcluster)  [unwired: 13 in]
  n106 = call <vilib>:"Simple Error Handler.vi"("type of dialog (OK msg:1)"=w15, "error in (no error)"=w10) -> ()  [unwired: 3 in, 5 out]
  n107 = call <vilib>:"DAQmx Clear Task.vi"("task in"=w5, "error in"=w2) -> ("error out"=w13:errorcluster)  [unwired: 13 in]
  n108 = call <vilib>:"Simple Error Handler.vi"("type of dialog (OK msg:1)"=w14, "error in (no error)"=w13) -> ()  [unwired: 3 in, 5 out]
  n109 = while {
    stop <- w266 stop-if-true
    # "Debug here"
    # "Hack to make looping work"
    # "start only when\nthere is  a connection"
    # "TCP data output"
    n110 = Wait (ms)(milliseconds to wait=u32 0) -> ()  [unwired: 1 out]
    n111 = call <vilib>:"TCP Listen.vi"("timeout ms (wait forever: -1)"=500, "port"="TCP data out port") -> ("error out"=w267:errorcluster, "connection ID"=w268:refnum<k5>)  [unwired: 5 in, 3 out]
    n112 = Unbundle By Name(w267) -> ("status"=w263:bool)
    n113 = Not(x=w263) -> (.not. x?=w262:bool)
    n114 = case shown="True" w262 {
      tunnel: w268 -> [_ w274]
      tunnel: w267 -> [_ w273]
      frame False {
        # "closing connection cannot happen as it was not openned"
        # "do nothing"
      }
      frame True {
        n115 = while {
          tunnel: w274 -> [w291]
          tunnel: [w290] -> w271
          shift-right: [w284] -> w272
          shift-left: w273 -> [w289]
          stop <- w285 stop-if-true
          # "Transmit only if it was not transmited before"
          # "Send data"
          n116 = local read "Last Transmited Loop Id"() -> (w288:i32)
          n117 = local read "Read Loop Id"() -> (w286:i32)
          n118 = Less?(x=w288, y=w286) -> (x < y?=w287:bool)
          n119 = local read "Closing Program"() -> (w283:bool)
          n120 = case shown="True" w287 {
            tunnel: w291 -> [w292 w306]
            tunnel: [w292 w305] -> w290
            tunnel: w289 -> [w293 w303]
            tunnel: [w293 w304] -> w284
            tunnel: w286 -> [_ w296]
            frame False {
            }
            frame True {
              # "discoonected\nfor testing"
              n121 = local read "IV read duration (ms)"() -> (w294:dbl)
              n122 = local read "Cuurent and Voltage"() -> (w297:waveform(dbl)[])
              n123 = local read "DC Voltage"() -> (w302:dbl)
              n124 = local read "AC Current"() -> (w299:dbl)
              n125 = local read "AC Voltage"() -> (w301:dbl)
              n126 = local read "DC Current"() -> (w300:dbl)
              n127 = local read "phase difference"() -> (w298:dbl)
              n128 = Index Array(array=w297) -> ()  [unwired: 2 in, 2 out]
              n129 = call "ADC to JSON.vi"("dt"=w294, "Phase"=w298, "LoopId"=w296, "I_AC"=w299, "I_DC"=w300, "U_AC"=w301, "U_DC"=w302) -> ("JSON"=w295:string)  [unwired: 3 in, 1 out]
              n130 = TCP Write(connection ID=w306, data in=w295, error in (no error)=w303) -> (connection ID out=w305:refnum<k5>, error out=w304:errorcluster)  [unwired: 1 in, 1 out]
              "Last Transmited Loop Id" <- w296
            }
          }
          n131 = Unbundle By Name(w284) -> ("code"=w275:i32)
          n132 = Equal?(x=56, y=w275) -> (x = y?=w281:bool)
          n133 = Equal?(x=66, y=w275) -> (x = y?=w280:bool)
          n134 = Equal?(x=52, y=w275) -> (x = y?=w276:bool)
          n135 = Compound Arithmetic op=OR(w281, w280, w276) -> (w282:bool)
          n136 = Or(x=w283, y=w282) -> (x .or. y?=w285:bool)
        }
        n137 = local write "TCP ADC"(TRUE ("TCP")) -> ()
        n138 = TCP Close Connection(connection ID=w271, error in (no error)=w272) -> ()  [unwired: 1 in, 2 out]
      }
    }
    n139 = local read "Closing Program"() -> (w266:bool)
    "TCP ADC" <- FALSE ("TCP")
  }
  n140 = while {
    stop <- w312 stop-if-true
    # "start only when\nthere is  a connection"
    # "Hack to make\nlooping work"
    # "TCP Incomming Commands"
    n141 = Wait (ms)(milliseconds to wait=u32 0) -> ()  [unwired: 1 out]
    n142 = call <vilib>:"TCP Listen.vi"("timeout ms (wait forever: -1)"=500, "port"="TCP command in port") -> ("error out"=w309:errorcluster, "connection ID"=w310:refnum<k5>)  [unwired: 5 in, 3 out]
    n143 = Unbundle By Name(w309) -> ("status"=w307:bool)
    n144 = Not(x=w307) -> (.not. x?=w308:bool)
    n145 = case shown="True" w308 {
      tunnel: w310 -> [_ w318]
      tunnel: w309 -> [_ w319]
      frame False {
      }
      frame True {
        n146 = while {
          tunnel: w319 -> [w329]
          tunnel: w318 -> [w330]
          tunnel: [w333] -> w317
          tunnel: [w332] -> w316
          stop <- w341 stop-if-true
          # "improve this by adding separate flag"
          # "Errors if connection was lost"
          # "Timeout"
          # "check if connected\nto the server"
          n147 = call "TCP Read.vi"("error in (no error)"=w329, "TCP Network Connection in"=w330) -> ("error out"=w327:errorcluster, "Message data out"=w323:string, "TCP Network Connection out"=w328:refnum<k5>)  [unwired: 7 in]
          n148 = Unbundle By Name(w327) -> ("code"=w334:i32)
          n149 = Wait (ms)(milliseconds to wait=u32 0) -> ()  [unwired: 1 out]
          n150 = Equal?(x="", y=w323) -> (x = y?=w321:bool)
          n151 = Equal?(x=w334, y=52) -> (x = y?=w337:bool)
          n152 = Equal?(x=56, y=w334) -> (x = y?=w324:bool)
          n153 = Equal?(x=66, y=w334) -> (x = y?=w340:bool)
          n154 = Compound Arithmetic op=OR(w340, w337) -> (w325:bool)
          n155 = Compound Arithmetic op=OR(w321, w324, w325) -> (invert w326:bool)
          n156 = case shown="True" w326 {
            tunnel: w328 -> [w343 w350]
            tunnel: w327 -> [w342 w351]
            tunnel: [w343 w353] -> w333
            tunnel: [w342 w352] -> w332
            tunnel: w323 -> [_ w347]
            frame False {
            }
            frame True {
              # "Lock and respond upon execution model"
              n157 = call "JSON command parser.vi"("JSON command"=w347) -> ("Value"=w348:dbl, "Command string"=w349:string)  [unwired: 9 in]
              n158 = case shown="\"pulse\"" w349 {
                selector: w349 -> [w355 _ _ _ _ _ _]
                tunnel: w348 -> [_ _ w361 w363 w367 w374 w377]
                tunnel: ["ERROR" "OK" "OK" "OK" "OK" "OK" "OK"] -> w344
                frame "False", Default {
                  # "Unknown command"
                  n159 = Concatenate Strings("Recieved an unkown TCP command: " ("message"), w355) -> (w357:string)
                  n160 = One Button Dialog(message=w357) -> ()  [unwired: 1 in, 1 out]
                }
                frame "pulse" {
                  n161 = local write "Pulse"(TRUE ("Pulse")) -> ()
                }
                frame "dc_v" {
                  # "set DC voltage"
                  n162 = local write "V_out"(w361) -> ()
                }
                frame "ac_v" {
                  # "Set AC voltage amplitude"
                  n163 = local read "Oscilator\nSettings"() -> (w365:T2)
                  n164 = Bundle By Name(cluster=w365, "Amplitude"=w363) -> (w364:T2)
                  n165 = local write "Oscilator\nSettings"(w364) -> ()
                }
                frame "ac_frequency" {
                  n166 = local read "Oscilator\nSettings"() -> (w369:T2)
                  n167 = Bundle By Name(cluster=w369, "Frequency"=w367) -> (w368:T2)
                  n168 = local write "Oscilator\nSettings"(w368) -> ()
                }
                frame "ac" {
                  n169 = To Long Integer(number=w374) -> (32bit integer=w373:i32)
                  n170 = Equal To 0?(x=w373) -> (x = 0?=w372:bool)
                  n171 = Not(x=w372) -> (.not. x?=w371:bool)
                  n172 = local write "Wave On/Off"(w371) -> ()
                }
                frame "electrode_mode" {
                  # "0 = imaging\n1 = deposition"
                  n173 = To Long Integer(number=w377) -> (32bit integer=w379:i32)
                  n174 = Equal To 0?(x=w379) -> (x = 0?=w378:bool)
                  n175 = Not(x=w378) -> (.not. x?=w376:bool)
                  n176 = local write "Electrode mode"(w376) -> ()
                }
              }
              n177 = Concatenate Strings(w344, "\n") -> (w346:string)
              n178 = TCP Write(connection ID=w350, data in=w346, error in (no error)=w351) -> (connection ID out=w353:refnum<k5>, error out=w352:errorcluster)  [unwired: 1 in, 1 out]
              "External Command" <- w347
            }
          }
          n179 = local read "Closing Program"() -> (w339:bool)
          n180 = Or(x=w325, y=w339) -> (x .or. y?=w341:bool)
        }
        n181 = local write "TCP Control"(TRUE ("TCP Control")) -> ()
        n182 = TCP Close Connection(connection ID=w317, error in (no error)=w316) -> ()  [unwired: 1 in, 2 out]
      }
    }
    n183 = local read "Closing Program"() -> (w312:bool)
    "TCP Control" <- FALSE ("TCP")
  }
